vi "ReadbyWeakRefNumV2.vi"(8 "error in":errorcluster caption="entrée d'erreur", 11 "Control Ref":refnum<vi>) -> (0 "error out":errorcluster caption="sortie d'erreur", 3 "Valeur":variant)   [LabVIEW 2010]
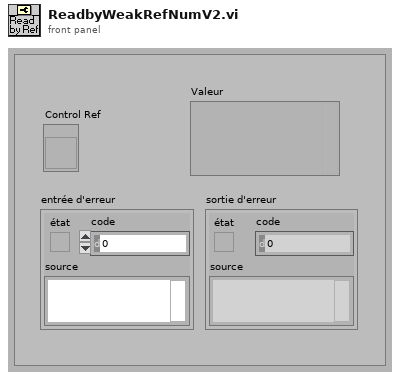
[diagram p1: front panel]
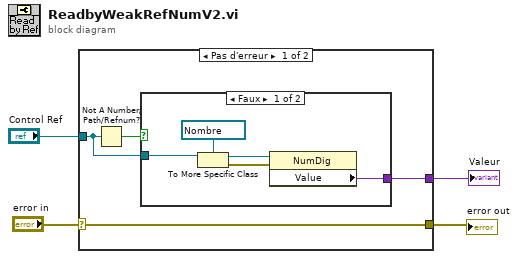
[diagram p0: block diagram]
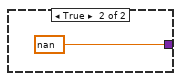
[diagram p2: hidden frame]
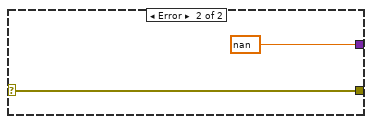
[diagram p3: hidden frame]
diagram:
  n1 = case shown="Pas d'erreur" "error in" {
    selector: "error in" -> [w5 w16]
    tunnel: "Control Ref" -> [w7 _]
    tunnel: [w6 nan ("Value")] -> w3
    tunnel: [w5 w16] -> w1
    frame No Error {
      n2 = Not A Number/Path/Refnum?(number/path/refnum=w7) -> (NaN/Path/Refnum?=w8:bool)
      n3 = case shown="Faux" w8 {
        tunnel: w7 -> [w9 _]
        tunnel: [w13 nan ("Value")] -> w6
        frame False {
          n4 = To More Specific Class(target class=refnum<vi> refnum ("référence"), reference=w9) -> (specific class reference=w11:refnum<vi>, error out=w10:errorcluster)  [unwired: 1 in]
          n5 = property class="NumDig"(reference=w11, error in=w10) -> ("Value"=w13:variant)  [unwired: 2 out]
        }
        frame True {
        }
      }
    }
    frame Error {
    }
  }
  "Valeur" <- w3
  "error out" <- w1
